vi "Scope.vi"(8 "error in (no error)":errorcluster, 9 "Timebase (0.005 s)":dbl=5e-09, 10 "Measurement Function (0: Rise Time)":i32(ring)=2 items=["Rise Time", "Fall Time", "Frequency", "Period", "Voltage RMS(AC)", "Voltage RMS(DC)", "Voltage RMS (AC,cycle)", "Voltage RMS (DC,cycle)", "Voltage Max", "Voltage Min", "Voltage Middle", "Voltage Vpp", "Voltage High", "Voltage Low", "Voltage Average", "Voltage Average (cycle)", "Width Negative", "Width Positive", "Duty Cycle Positive", "Amplitude", "Overshoot", "Preshoot", "Voltage Base", "Voltage Upper", "Time Max", "Time Min", "Color Grade Crossing", "Color Grade Eye Width", "Color Grade Eye Height", "Color Grade Eye Q-Factory", "Color Grade Eye Duty Cycle Distortion(Percent)", "Color Grade Eye Duty Cycle Distortion(Time)", "Color Grade Eye Jitter(PP)", "Color Grade Eye Width(RMS)", "Cycle-cycle Duty Jitter(Rising)", "Cycle-cycle Duty Jitter(Falling)", "Cycle-cycle Jitter(Rising)", "Cycle-cycle Jitter(Falling)", "Cycle-cycle - Width", "Cycle-cycle + Width", "Date Rate", "Unit Interval", "FFT Delta Frequency", "FFT Delta Magnitude", "FFT Frequency", "FFT Magnitude", "Slew Rate", "Area (Entire Display)", "Area(Single Cycle)", "Duty Cycle (Rising)", "Duty Cycle (Falling)"], 11 "Channel (1: Channel 1)":i32(ring)=1 items=["Channel 1"=1, "Channel 2"=2, "Channel 3"=3, "Channel 4"=4]) -> (0 "error out":errorcluster, 3 "Measurement":dbl)   [LabVIEW 2011]
doc: "This VI autoscales a selected Agilent Scope Channel, sets the trigger at 50%, and takes the measurement selected.\n\nInputs:\n1. Channel: The scope channel to view/measure on the scope.\n2. Mesaurement Function: The measurement to take (if desired). (Frequency, Duty Cycle, etc.)\n3. Timebase: The horizontal time scale of the scope. (5ns, 10ms, etc.)\n\nOutputs:\n1. Measurement: The result of the scope measurement selected."
uses:
  <instrlib>/Agilent 8000 Series/Public/Data/Low Level/Fetch Measurement (More).vi
  <instrlib>/Agilent 8000 Series/Public/Configure/Configure Trigger (Edge).vi
  <instrlib>/Agilent 8000 Series/Public/Data/Read Measurement (More).vi
  <instrlib>/Agilent 8000 Series/Agilent 8000 Series.lvlib
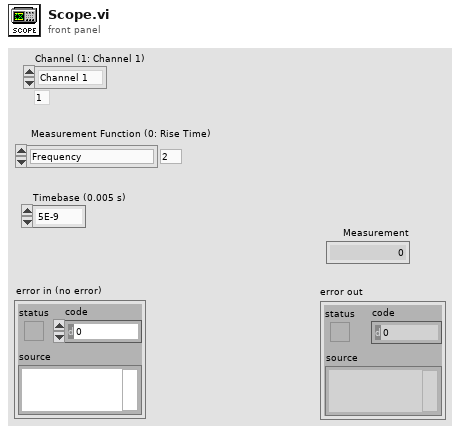
[diagram p1: front panel]
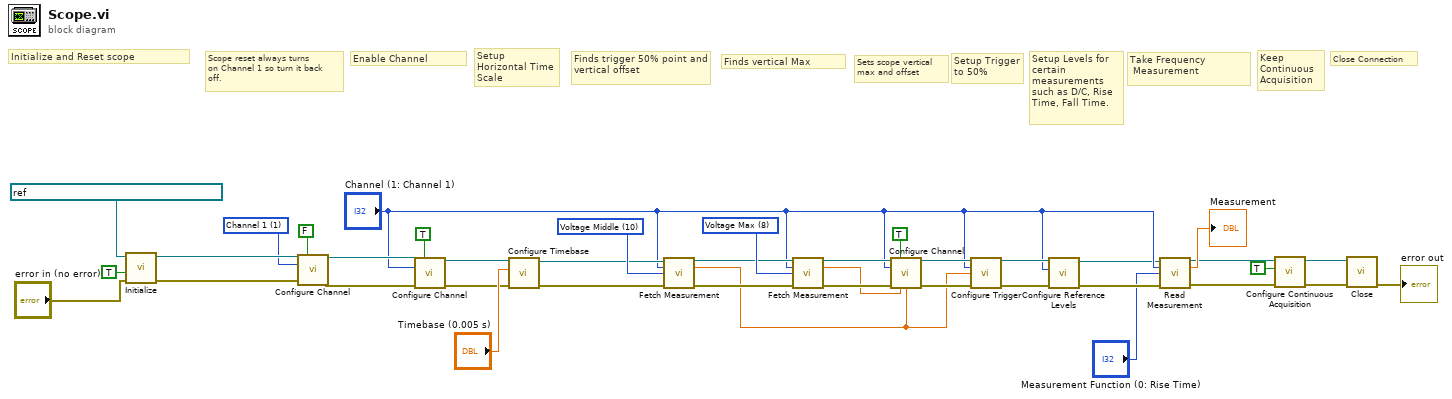
[diagram p0: block diagram]
diagram:
  w7 = 1 items=["Channel 1"=1, "Channel 2"=2, "Channel 3"=3, "Channel 4"=4] ("Channel (1: Channel 1)")
  w22 = 8 items=["Rise Time", "Fall Time", "Frequency", "Period", "Voltage RMS(AC)", "Voltage RMS(DC)", "Voltage RMS (AC,cycle)", "Voltage RMS (DC,cycle)", "Voltage Max", "Voltage Min", "Voltage Middle", "Voltage Vpp", "Voltage High", "Voltage Low", "Voltage Average", "Voltage Average (cycle)", "Width Negative", "Width Positive", "Duty Cycle Positive", "Amplitude", "Overshoot", "Preshoot", "Voltage Base", "Voltage Upper", "Time Max", "Time Min", "Color Grade Crossing", "Color Grade Eye Width", "Color Grade Eye Height", "Color Grade Eye Q-Factory", "Color Grade Eye Duty Cycle Distortion(Percent)", "Color Grade Eye Duty Cycle Distortion(Time)", "Color Grade Eye Jitter(PP)", "Color Grade Eye Width(RMS)", "Cycle-cycle Duty Jitter(Rising)", "Cycle-cycle Duty Jitter(Falling)", "Cycle-cycle Jitter(Rising)", "Cycle-cycle Jitter(Falling)", "Cycle-cycle - Width", "Cycle-cycle + Width", "Date Rate", "Unit Interval", "FFT Delta Frequency", "FFT Delta Magnitude", "FFT Frequency", "FFT Magnitude", "Slew Rate", "Area (Entire Display)", "Area(Single Cycle)", "Duty Cycle (Rising)", "Duty Cycle (Falling)"] ("Measurement Function (0: Rise Time)")
  w25 = 10 items=["Rise Time", "Fall Time", "Frequency", "Period", "Voltage RMS(AC)", "Voltage RMS(DC)", "Voltage RMS (AC,cycle)", "Voltage RMS (DC,cycle)", "Voltage Max", "Voltage Min", "Voltage Middle", "Voltage Vpp", "Voltage High", "Voltage Low", "Voltage Average", "Voltage Average (cycle)", "Width Negative", "Width Positive", "Duty Cycle Positive", "Amplitude", "Overshoot", "Preshoot", "Voltage Base", "Voltage Upper", "Time Max", "Time Min", "Color Grade Crossing", "Color Grade Eye Width", "Color Grade Eye Height", "Color Grade Eye Q-Factory", "Color Grade Eye Duty Cycle Distortion(Percent)", "Color Grade Eye Duty Cycle Distortion(Time)", "Color Grade Eye Jitter(PP)", "Color Grade Eye Width(RMS)", "Cycle-cycle Duty Jitter(Rising)", "Cycle-cycle Duty Jitter(Falling)", "Cycle-cycle Jitter(Rising)", "Cycle-cycle Jitter(Falling)", "Cycle-cycle - Width", "Cycle-cycle + Width", "Date Rate", "Unit Interval", "FFT Delta Frequency", "FFT Delta Magnitude", "FFT Frequency", "FFT Magnitude", "Slew Rate", "Area (Entire Display)", "Area(Single Cycle)", "Duty Cycle (Rising)", "Duty Cycle (Falling)"] ("Measurement Function (0: Rise Time)")
  # "Scope reset always turns\non Channel 1 so turn it back\noff."
  # "Close Connection"
  # "Sets scope vertical\nmax and offset"
  # "Finds vertical Max"
  # "Finds trigger 50% point and vertical offset"
  # "Enable Channel"
  # "Keep\nContinuous\nAcquisition"
  # "Initialize and Reset scope"
  # "Setup Levels for\ncertain measurements such as D/C, Rise Time, Fall Time."
  # "Setup Trigger to 50%"
  # "Take Frequency\n Measurement"
  # "Setup Horizontal Time Scale"
  n1 = call <instrlib>:"Initialize.vi"("error in (no error)"="error in (no error)", "Reset (True)"=TRUE, "VISA resource name"=refnum<visa-resource-name> "TCPIP0::192.168.1.130::inst0::INSTR") -> ("error out"=w8:errorcluster, "VISA resource name out"=w9:refnum<visa-resource-name>)  [unwired: 7 in]
  n2 = call <instrlib>:"Configure Channel.vi"("VISA resource name"=w9, "Enable Channel (Enable)"=FALSE, "Channel (1: Channel 1)"=w7, "error in (no error)"=w8) -> ("VISA resource name out"=w11:refnum<visa-resource-name>, "error out"=w10:errorcluster)  [unwired: 10 in]
  n3 = call <instrlib>:"Configure Channel.vi"("VISA resource name"=w11, "Enable Channel (Enable)"=TRUE, "Channel (1: Channel 1)"="Channel (1: Channel 1)", "error in (no error)"=w10) -> ("VISA resource name out"=w29:refnum<visa-resource-name>, "error out"=w28:errorcluster)  [unwired: 10 in]
  n4 = call <instrlib>:"Configure Timebase.vi"("error in (no error)"=w28, "Timebase (0.005 s)"="Timebase (0.005 s)", "VISA resource name"=w29) -> ("error out"=w23:errorcluster, "VISA resource name out"=w24:refnum<visa-resource-name>)  [unwired: 7 in]
  n5 = call-poly <instrlib>:"Fetch Measurement.vi"("VISA resource name"=w24, "Channel (1: Channel 1)"="Channel (1: Channel 1)", "Measurement Function (0: Rise Time)"=w25, "error in (no error)"=w23) -> ("VISA resource name out"=w21:refnum<visa-resource-name>, "Measurement"=w13:dbl, "error out"=w20:errorcluster)  [unwired: 9 in]
  n6 = call-poly <instrlib>:"Fetch Measurement.vi"("VISA resource name"=w21, "Channel (1: Channel 1)"="Channel (1: Channel 1)", "Measurement Function (0: Rise Time)"=w22, "error in (no error)"=w20) -> ("VISA resource name out"=w18:refnum<visa-resource-name>, "Measurement"=w14:dbl, "error out"=w15:errorcluster)  [unwired: 9 in]
  n7 = call <instrlib>:"Configure Channel.vi"("VISA resource name"=w18, "Enable Channel (Enable)"=TRUE, "Channel (1: Channel 1)"="Channel (1: Channel 1)", "error in (no error)"=w15, "Vertical Range (2.0 V)"=w14, "Vertical Offset (0.0 V)"=w13) -> ("VISA resource name out"=w17:refnum<visa-resource-name>, "error out"=w16:errorcluster)  [unwired: 8 in]
  n8 = call-poly <instrlib>:"Configure Trigger.vi"("VISA resource name"=w17, "Trigger Source (1: Channel 1)"="Channel (1: Channel 1)", "Trigger Level (0.0 V)"=w13, "error in (no error)"=w16) -> ("VISA resource name out"=w5:refnum<visa-resource-name>, "error out"=w6:errorcluster)  [unwired: 10 in]
  n9 = call <instrlib>:"Configure Reference Levels.vi"("error in (no error)"=w6, "Channel (31: All Waveforms)"="Channel (1: Channel 1)", "VISA resource name"=w5) -> ("error out"=w3:errorcluster, "VISA resource name out"=w2:refnum<visa-resource-name>)  [unwired: 7 in]
  n10 = call-poly <instrlib>:"Read Measurement.vi"("VISA resource name"=w2, "Channel (1: Channel 1)"="Channel (1: Channel 1)", "Measurement Function (0: Rise Time)"="Measurement Function (0: Rise Time)", "error in (no error)"=w3) -> ("VISA resource name out"=w34:refnum<visa-resource-name>, "Measurement"=→"Measurement":dbl, "error out"=w33:errorcluster)  [unwired: 9 in]
  n11 = call <instrlib>:"Configure Continuous Acquisition.vi"("error in (no error)"=w33, "Enable Continuous Acquisition Mode (T:Enable)"=TRUE, "VISA resource name"=w34) -> ("error out"=w31:errorcluster, "VISA resource name out"=w32:refnum<visa-resource-name>)  [unwired: 7 in]
  n12 = call <instrlib>:"Close.vi"("error in (no error)"=w31, "VISA resource name"=w32) -> ("error out"=→"error out":errorcluster)  [unwired: 9 in]
